vi "Image Merge Axes v10.5.1.vi"(0 "Image In":dbl[][](array[numeric]), 9 "CCD Area Format":T1) -> (4 "Image Out":dbl[][](array[numeric]))   [LabVIEW 2010]
uses:
  Symphony/TypeDefs/Symphony Area Format.ctl
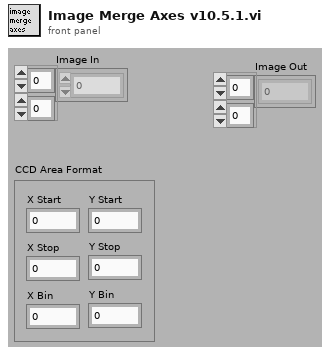
[diagram p1: front panel]
types:
  T1 = typedef "Symphony Area Format.ctl" = cluster{"XStart":i32, "YStart":i32, "XStop":i32, "YStop":i32, "XBin":i32, "YBin":i32}
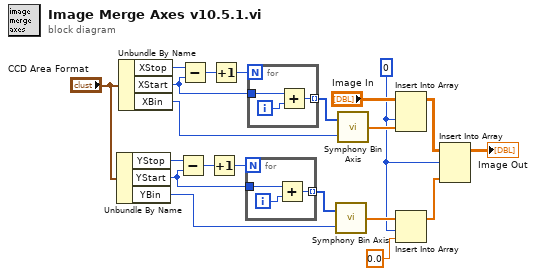
[diagram p0: block diagram]
diagram:
  w1 = 0 ("index (row)")
  n1 = Unbundle By Name("CCD Area Format") -> ("YStop"=w14:i32, "YStart"=w13:i32, "YBin"=w7:i32)
  n2 = Unbundle By Name("CCD Area Format") -> ("XStop"=w18:i32, "XStart"=w17:i32, "XBin"=w10:i32)
  n3 = Subtract(x=w14, y=w13) -> (x-y=w16:i32)
  n4 = Subtract(x=w18, y=w17) -> (x-y=w20:i32)
  n5 = Increment(x=w16) -> (x+1=w15:i32)
  n6 = Increment(x=w20) -> (x+1=w19:i32)
  n7 = for {
    N: w15 -> [_]
    tunnel: w13 -> [w23]
    tunnel: [w22] -> w8 mode=indexing
    i -> [w24]
    n8 = Add(x=w23, y=w24) -> (x+y=w22:i32)
  }
  n9 = for {
    N: w19 -> [_]
    tunnel: w17 -> [w26]
    tunnel: [w25] -> w11 mode=indexing
    i -> [w27]
    n10 = Add(x=w26, y=w27) -> (x+y=w25:i32)
  }
  n11 = call "Symphony Bin Axis.vi"("Binning Factor"=w7, "Axis In"=w8) -> ("Axis Out"=w6:dbl[])
  n12 = call "Symphony Bin Axis.vi"("Binning Factor"=w10, "Axis In"=w11) -> ("Axis Out"=w9:dbl[])
  n13 = Insert Into Array(array="Image In", index (col)=w1, new element=w9) -> (w21:dbl[][])  [unwired: 1 in]
  n14 = Insert Into Array(array=w6, index=w1, new element=0.0 ("new element/subarray")) -> (w4:dbl[])
  n15 = Insert Into Array(array=w21, index (row)=w1, new element=w4) -> (→"Image Out":dbl[][])  [unwired: 1 in]
